vi "DiffRobot.vi"() -> ()   [LabVIEW 2023]
doc: "Manually blink and LED attached to a digital output channel of a LINX device by clicking and LED control in LabVIEW."
uses:
  <vilib>/Instr/_visa.llb/VISA Configure Serial Port (Instr).vi
  <vilib>/MakerHub/Xbox-One-Controller/Public/Open First Controller.vi
  <vilib>/MakerHub/Xbox-One-Controller/LMH-Xbox-One-Controller.lvlib
panel:
  out "Boolean":bool
  out "Distance":dbl
  in  "stop":bool
  out "omega":dbl
  out "V":dbl
  in  "Arduino COM":refnum<visa-resource-name>
  out "Serial Send:":string
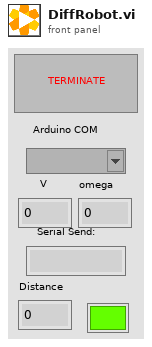
[diagram p1: front panel]
types:
  T1 = typedef "LMH-Xbox-One-Controller.lvlib/Xbox One Controller Ref.ctl" = cluster{"Controller Ref":refnum<k1>, "Event Refnum":refnum<event-registration>, "Worker Ref":refnum<vi>}
  T2 = typedef "LMH-Xbox-One-Controller.lvlib/All Axis Data.ctl" = cluster{"Left Stick":cluster{"X Axis":i32, "Y Axis":i32}, "Right Stick":cluster{"X Axis":i32, "Y Axis":i32}, "Triggers":i32, "D-Pad":T3}
  T3 = typedef "LMH-Xbox-One-Controller.lvlib/DPad Enum.ctl" = enum16{"Idle", "Up", "Up / Right", "Right", "Down / Right", "Down", "Down / Left", "Left", "Up / Left"}
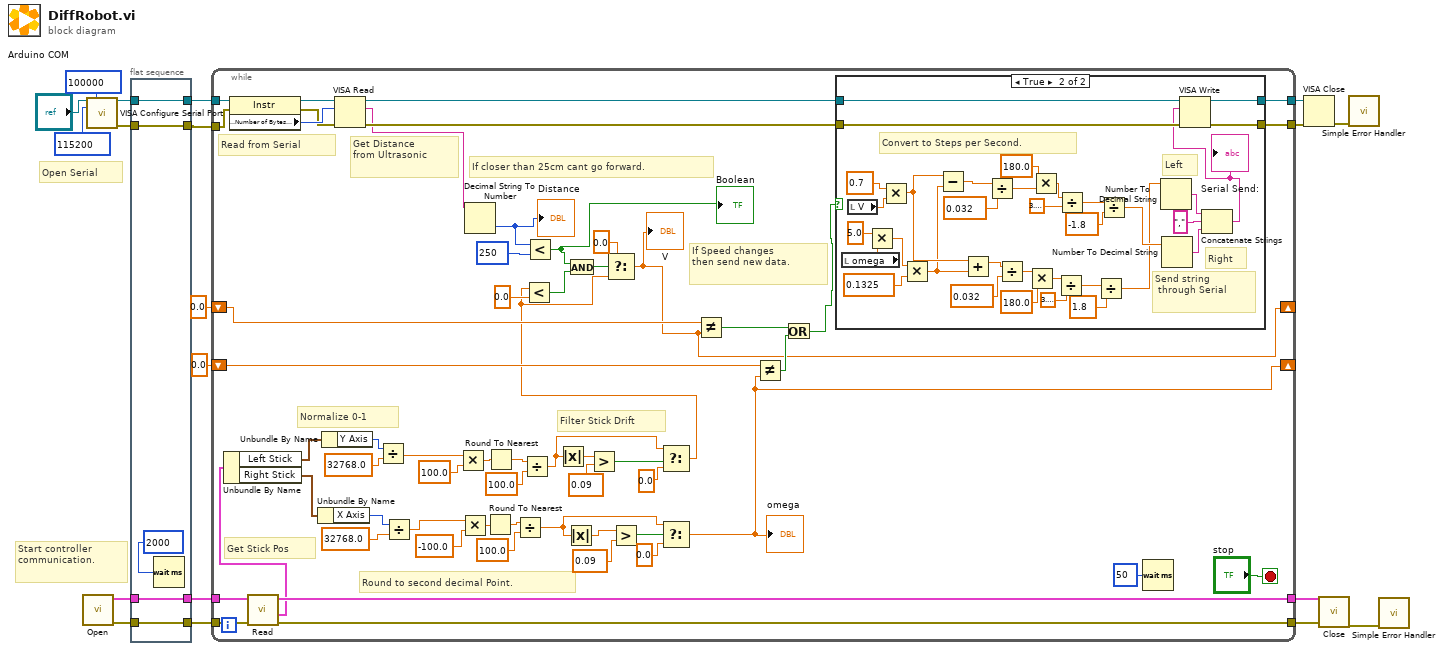
[diagram p0: block diagram]
diagram:
  # "Start controller\ncommunication."
  # "Open Serial"
  n1 = call-poly <vilib>:"Open.vi"() -> ("Error Out"=w3:errorcluster, "Xbox One Controller"=w4:T1)  [unwired: 9 in, 1 out]
  n2 = call-poly "VISA Configure Serial Port"("VISA resource name"="Arduino COM", "timeout (10sec)"=u32 100000, "baud rate (9600)"=u32 115200) -> ("VISA resource name out"=w15:refnum<visa-resource-name>, "error out"=w13:errorcluster)  [unwired: 11 in]
  n3 = flat-sequence {
    tunnel: [w23] -> w16
    tunnel: w15 -> [w23]
    tunnel: [w22] -> w14
    tunnel: w13 -> [w22]
    tunnel: [w21] -> w11
    tunnel: w4 -> [w21]
    tunnel: [w20] -> w5
    tunnel: w3 -> [w20]
    frame #0 {
      n4 = Wait (ms)(milliseconds to wait=u32 2000) -> ()  [unwired: 1 out]
    }
  }
  n5 = while {
    tunnel: w16 -> [w82]
    tunnel: w14 -> [w81]
    shift-right: [w26] -> _
    shift-left: 0.0 ("V") -> [w40]
    shift-right: [w36] -> _
    shift-left: 0.0 ("omega") -> [w39]
    tunnel: w5 -> [w56]
    tunnel: w11 -> [w55]
    tunnel: [w53] -> w9
    tunnel: [w52] -> w8
    tunnel: [w31] -> w2
    tunnel: [w30] -> w1
    stop <- "stop" stop-if-true
    # "If Speed changes\nthen send new data."
    # "If closer than 25cm cant go forward."
    # "Get Distance\nfrom Ultrasonic"
    # "Read from Serial"
    # "Filter Stick Drift"
    # "Round to second decimal Point."
    # "Normalize 0-1"
    # "Get Stick Pos"
    n6 = property class="Instr"(reference=w82, error in=w81) -> (reference out=w79:refnum<visa-resource-name>, error out=w78:errorcluster, "Serial Settings:Number of Bytes at Serial Port"=w80:u32)
    n7 = call <vilib>:"Read.vi"("Error In"=w56, "Xbox One Controller Ref"=w55) -> ("Error Out"=w53:errorcluster, "All Axis"=w41:T2, "Xbox One Controller Ref"=w52:T1)  [unwired: 6 in, 1 out]
    n8 = Unbundle By Name(w41) -> ("Left Stick"=w47:cluster{"X Axis":i32, "Y Axis":i32}, "Right Stick"=w73:cluster{"X Axis":i32, "Y Axis":i32})
    n9 = Unbundle By Name(w73) -> ("X Axis"=w74:i32)
    n10 = Unbundle By Name(w47) -> ("Y Axis"=w46:i32)
    n11 = VISA Read(VISA resource name=w79, byte count=w80, error in (no error)=w78) -> (VISA resource name out=w77:refnum<visa-resource-name>, read buffer=w51:string, error out=w76:errorcluster)  [unwired: 1 out]
    n12 = Divide(x=w46, y=32768.0) -> (x/y=w44:dbl)
    n13 = Divide(x=w74, y=32768.0) -> (x/y=w70:dbl)
    n14 = Multiply(x=w44, y=100.0) -> (x*y=w68:dbl)
    n15 = Multiply(x=w70, y=-100.0) -> (x*y=w71:dbl)
    n16 = Decimal String To Number(string=w51) -> (number=w34:i32)  [unwired: 2 in, 1 out]
    "Distance" <- w34
    n17 = Round To Nearest(number=w71) -> (nearest integer value=w49:dbl)
    n18 = Round To Nearest(number=w68) -> (nearest integer value=w65:dbl)
    n19 = Divide(x=w49, y=100.0) -> (x/y=w67:dbl)
    n20 = Divide(x=w65, y=100.0) -> (x/y=w42:dbl)
    n21 = Less?(x=w34, y=250) -> (x < y?=w25:bool)
    "Boolean" <- w25
    n22 = Absolute Value(x=w42) -> (abs(x)=w72:dbl)
    n23 = Absolute Value(x=w67) -> (abs(x)=w48:dbl)
    n24 = Greater?(x=w72, y=0.09) -> (0:w69:bool)
    n25 = Greater?(x=w48, y=0.09) -> (0:w66:bool)
    n26 = Select(t=w42, s=w69, f=0.0) -> (s? t:f=w27:dbl)
    n27 = Less?(x=w27, y=0.0) -> (x < y?=w33:bool)
    n28 = And(x=w25, y=w33) -> (x .and. y?=w29:bool)
    n29 = Select(t=0.0, s=w29, f=w27) -> (s? t:f=w26:dbl)
    "V" <- w26
    n30 = Select(t=w67, s=w66, f=0.0) -> (s? t:f=w36:dbl)
    "omega" <- w36
    n31 = Not Equal?(x=w40, y=w26) -> (x != y?=w38:bool)
    n32 = Not Equal?(x=w39, y=w36) -> (x != y?=w37:bool)
    n33 = Or(x=w38, y=w37) -> (x .or. y?=w28:bool)
    n34 = case shown="True" w28 {
      tunnel: w77 -> [w84 w118]
      tunnel: w76 -> [w83 w117]
      tunnel: [w84 w92] -> w31
      tunnel: [w83 w91] -> w30
      frame False {
      }
      frame True {
        # "Send string\n through Serial"
        # "Left"
        # "Right"
        # "Convert to Steps per Second."
        n35 = local read "omega"() -> (w93:dbl)
        n36 = local read "V"() -> (w94:dbl)
        n37 = Multiply(x=5.0, y=w93) -> (x*y=w95:dbl)
        n38 = Multiply(x=0.7, y=w94) -> (x*y=w97:dbl)
        n39 = Multiply(x=w95, y=0.1325) -> (x*y=w85:dbl)
        n40 = Subtract(x=w97, y=w85) -> (x-y=w107:dbl)
        n41 = Add(x=w97, y=w85) -> (x+y=w86:dbl)
        n42 = Divide(x=w107, y=0.032) -> (x/y=w105:dbl)
        n43 = Divide(x=w86, y=0.032) -> (x/y=w113:dbl)
        n44 = Multiply(x=w113, y=180.0) -> (x*y=w111:dbl)
        n45 = Multiply(x=180.0, y=w105) -> (x*y=w103:dbl)
        n46 = Divide(x=w111, y=3.141592653589793) -> (x/y=w109:dbl)
        n47 = Divide(x=w103, y=3.141592653589793) -> (x/y=w102:dbl)
        n48 = Divide(x=w109, y=1.8) -> (x/y=w99:dbl)
        n49 = Divide(x=w102, y=-1.8) -> (x/y=w100:dbl)
        n50 = Number To Decimal String(number=w99) -> (decimal integer string=w116:string)  [unwired: 1 in]
        n51 = Number To Decimal String(number=w100) -> (decimal integer string=w115:string)  [unwired: 1 in]
        n52 = Concatenate Strings(w116, ",", w115) -> (w90:string)
        "Serial Send:" <- w90
        n53 = VISA Write(VISA resource name=w118, write buffer=w90, error in (no error)=w117) -> (VISA resource name out=w92:refnum<visa-resource-name>, error out=w91:errorcluster)  [unwired: 1 out]
      }
    }
    n54 = Wait (ms)(milliseconds to wait=u32 50) -> ()  [unwired: 1 out]
  }
  n55 = VISA Close(VISA resource name=w2, error in (no error)=w1) -> (error out=w12:errorcluster)
  n56 = call <vilib>:"Close.vi"("Error In"=w9, "Xbox One Controller Ref"=w8) -> ("Error Out"=w10:errorcluster)  [unwired: 9 in]
  n57 = call <vilib>:"Simple Error Handler.vi"("error in (no error)"=w12) -> ()  [unwired: 4 in, 5 out]
  n58 = call <vilib>:"Simple Error Handler.vi"("error in (no error)"=w10) -> ()  [unwired: 4 in, 5 out]
